vi "PartSetup.vi"(8 "error in (no error)":errorcluster) -> (0 "error out":errorcluster)   [LabVIEW 2015]
uses:
  Control 1.ctl
  Partsetup-Exit.ctl
  Partsetup-Delete.ctl
  Partsetup- Save.ctl
  <vilib>/addons/database/_DB Variant To Data/Database Variant To Data.xnode
  <vilib>/addons/database/NI_Database_API.lvlib
  <vilib>/addons/database/Connection.llb/DB Tools Open Connec (String).vi
  Galobal variable_TI.vi
panel:
  in  "Save":T1
  in  "Delete":T2
  in  "Exit":T3
  in  "Data Insert":variant
  in  "Existing Model Name":string(combo)
  in  "Part setup":T4
  # "UM"
  # "Atma Autotech Engineers Pvt.Ltd"
  # "PART SETUP"
  # "Existing Model Name"
  # "First motor testing Parameter"
  # "Printing Info"
  # "Second motor testing Parameter"
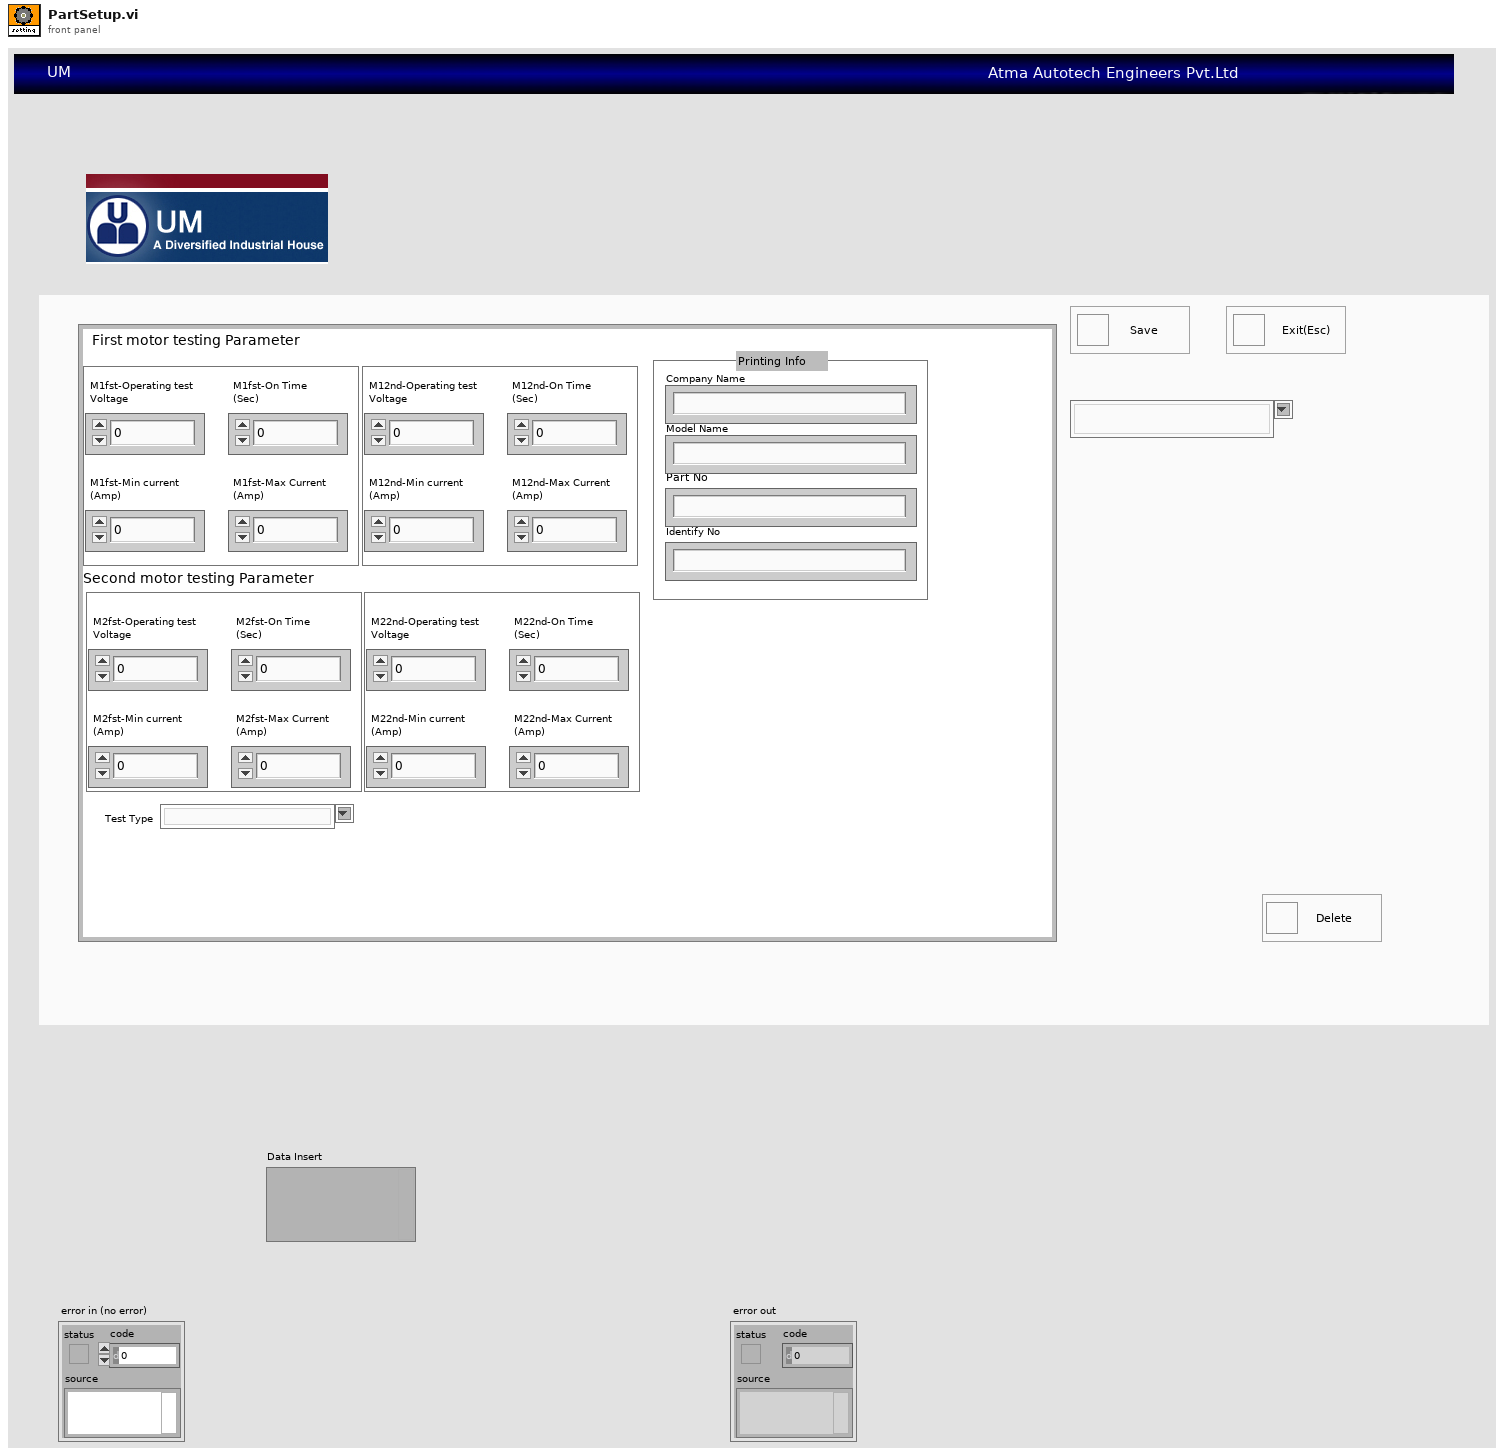
[diagram p1: front panel]
types:
  T1 = typedef "Partsetup- Save.ctl" = bool
  T2 = typedef "Partsetup-Delete.ctl" = bool
  T3 = typedef "Partsetup-Exit.ctl" = bool
  T4 = typedef "Control 1.ctl" = cluster{"Model Name":string, "Company Name":string, "Part No":string, "Identify No":string, "M1fst-Operating test\nVoltage":dbl, "M1fst-On Time \n(Sec)":dbl, "M1fst-Min current \n(Amp)":dbl, "M1fst-Max Current\n(Amp)":dbl, "M12nd-Operating test\nVoltage":dbl, "M12nd-On Time \n(Sec)":dbl, "M12nd-Min current \n(Amp)":dbl, "M12nd-Max Current\n(Amp)":dbl, "M2fst-Operating test\nVoltage":dbl, "M2fst-On Time \n(Sec)":dbl, "M2fst-Min current \n(Amp)":dbl, "M2fst-Max Current\n(Amp)":dbl, "M22nd-Operating test\nVoltage":dbl, "M22nd-On Time \n(Sec)":dbl, "M22nd-Min current \n(Amp)":dbl, "M22nd-Max Current\n(Amp)":dbl, "Test Type ":string}
  T5 = enum16{"New model Create", "Update", "DB-Read by condition", "DB-Read", "Delete"}
  T6 = typedef "NI_Database_API.lvlib/Conn ObjectReference.ctl" = refnum<k1>
  T7 = enum16{"Left Button", "Center Button", "Right Button", "Window Close"}
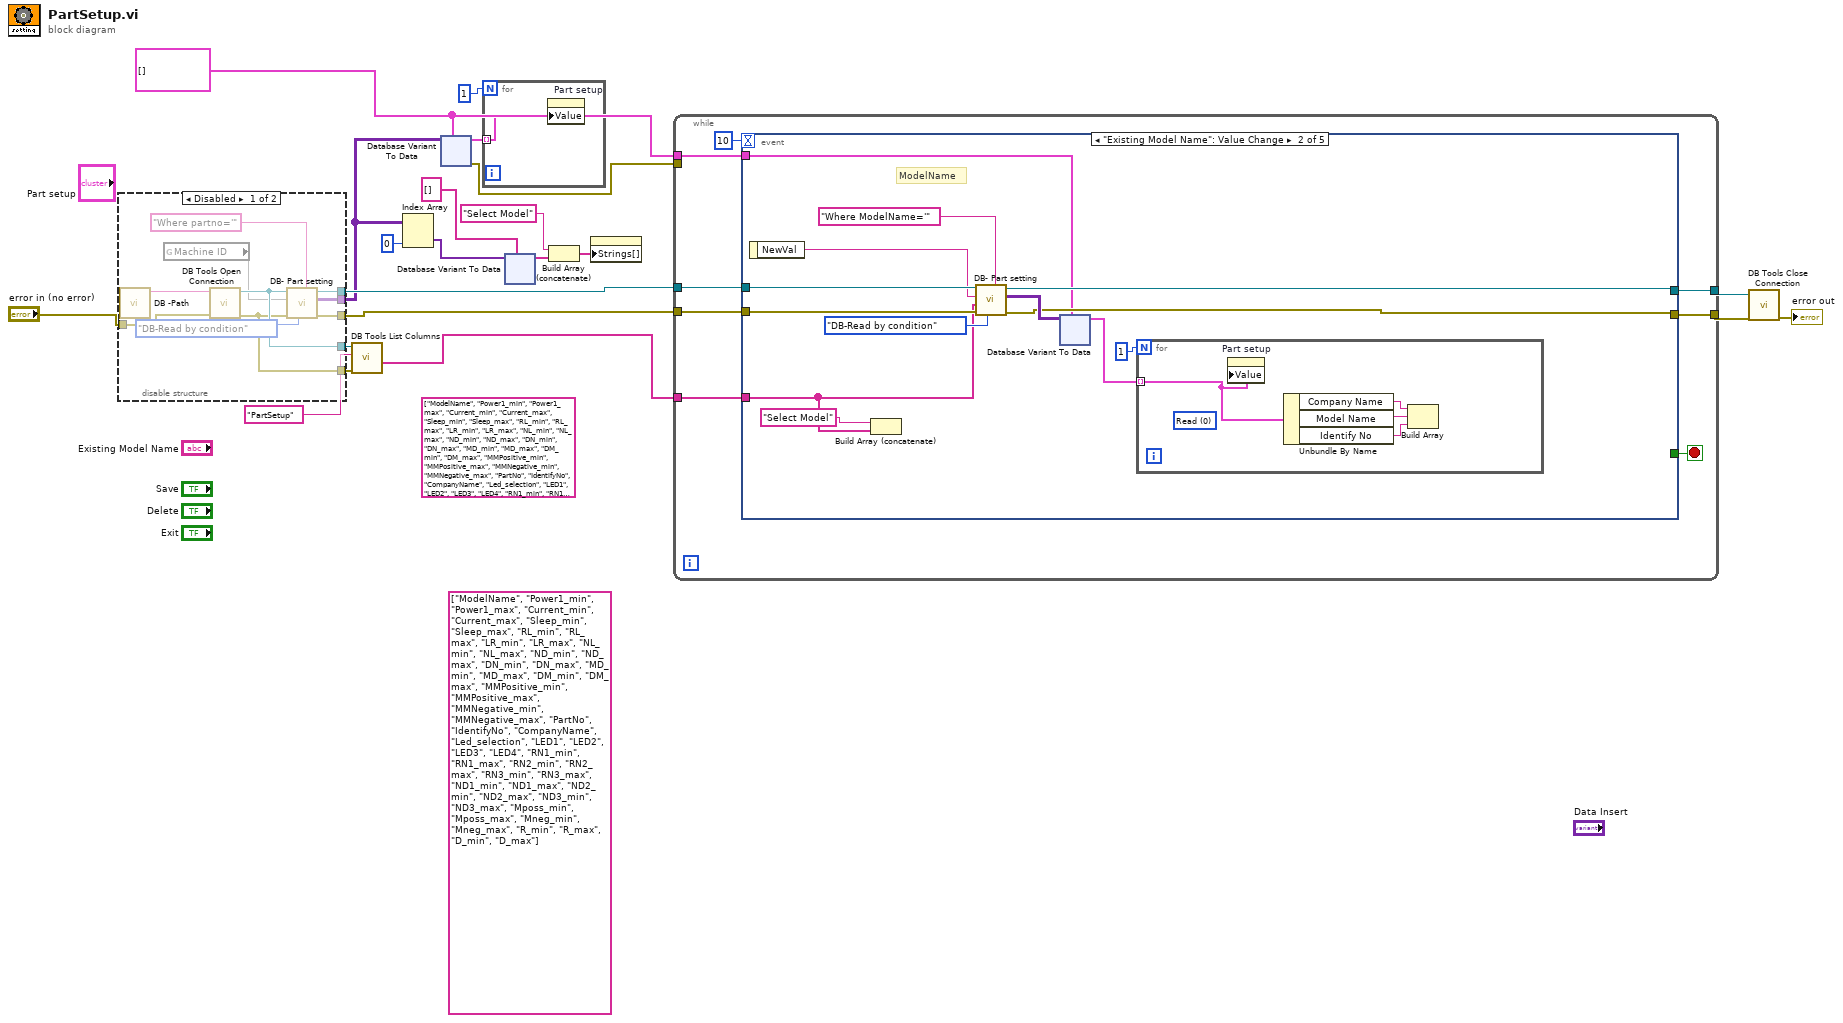
[diagram p0: block diagram]
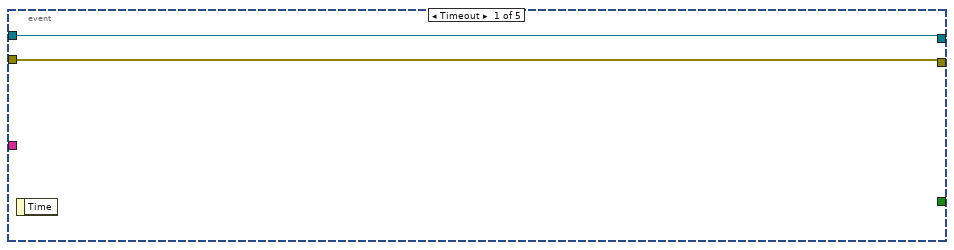
[diagram p3: hidden frame]
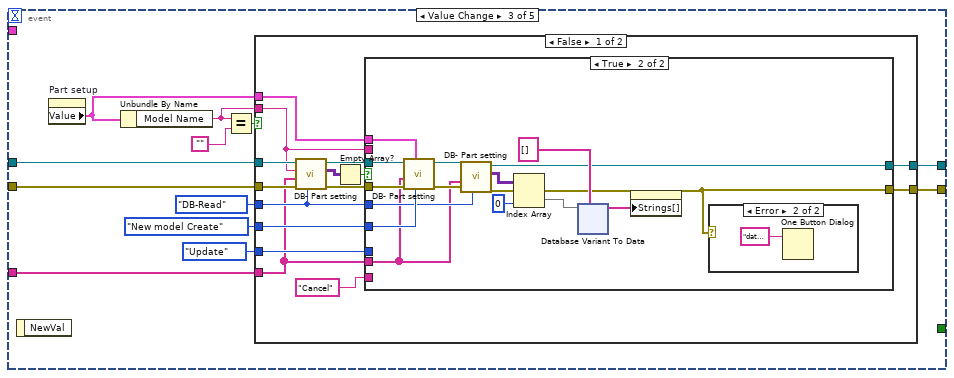
[diagram p4: hidden frame]
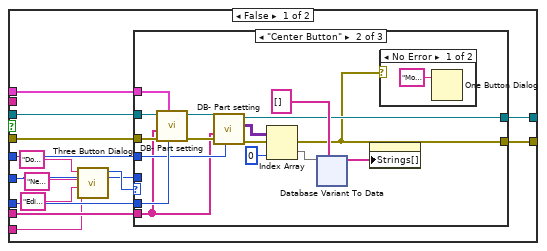
[diagram p5: hidden frame]
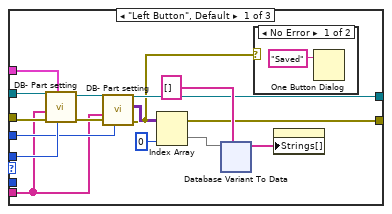
[diagram p6: hidden frame]
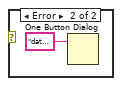
[diagram p7: hidden frame]
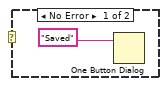
[diagram p10: hidden frame]
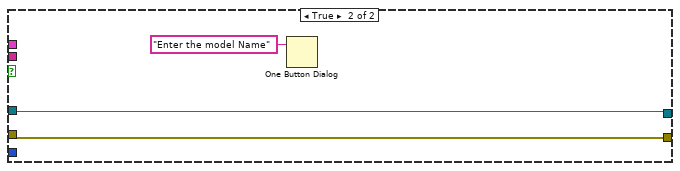
[diagram p11: hidden frame]
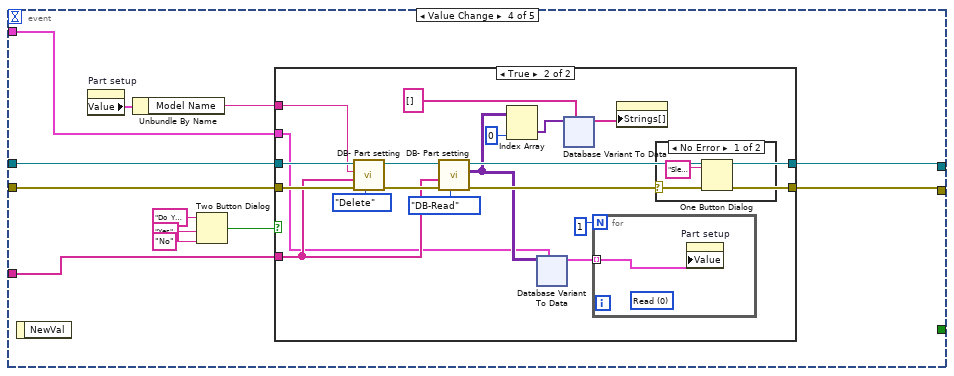
[diagram p12: hidden frame]
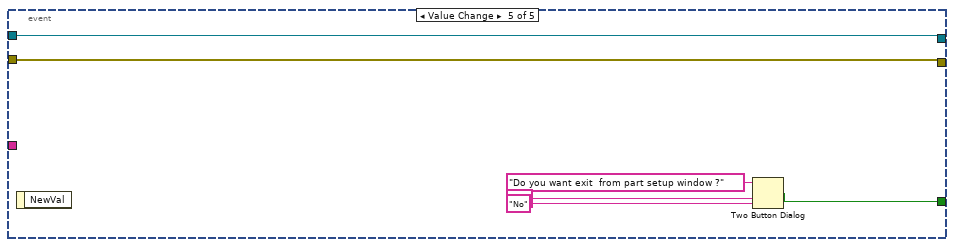
[diagram p15: hidden frame]
diagram:
  w4 = T4[] []
  (unwired) string[] ["ModelName", "Power1_min", "Power1_max", "Current_min", "Current_max", "Sleep_min", "Sleep_max", "RL_min", "RL_max", "LR_min", "LR_max", "NL_min", "NL_max", "ND_min", "ND_max", "DN_min", "DN_max", "MD_min", "MD_max", "DM_min", "DM_max", "MMPositive_min", "MMPositive_max", "MMNegative_min", "MMNegative_max", "PartNo", "IdentifyNo", "CompanyName", "Led_selection", "LED1", "LED2", "LED3", "LED4", "RN1_min", "RN1_max", "RN3_min", "RN3_max", "ND1_min", "ND1_max", "ND2_min", "ND2_max", "Mposs_min", "Mposs_max", "Mneg_min", "Mneg_max", "R_min", "R_max", "D_min", "D_max"] ("columns")
  (unwired) string[] ["ModelName", "Power1_min", "Power1_max", "Current_min", "Current_max", "Sleep_min", "Sleep_max", "RL_min", "RL_max", "LR_min", "LR_max", "NL_min", "NL_max", "ND_min", "ND_max", "DN_min", "DN_max", "MD_min", "MD_max", "DM_min", "DM_max", "MMPositive_min", "MMPositive_max", "MMNegative_min", "MMNegative_max", "PartNo", "IdentifyNo", "CompanyName", "Led_selection", "LED1", "LED2", "LED3", "LED4", "RN1_min", "RN1_max", "RN2_min", "RN2_max", "RN3_min", "RN3_max", "ND1_min", "ND1_max", "ND2_min", "ND2_max", "ND3_min", "ND3_max", "Mposs_min", "Mposs_max", "Mneg_min", "Mneg_max", "R_min", "R_max", "D_min", "D_max"] ("columnsName")
  n1 = disable-structure shown="Disabled" {
    disable-tunnel: "error in (no error)" -> [w30 _]
    disable-tunnel: [w29 _] -> w18
    disable-tunnel: [w28 _] -> w17
    disable-tunnel: [w26 _] -> w11
    disable-tunnel: [w25 _] -> w8
    disable-tunnel: [w24 _] -> w7
    frame Disabled {
      n2 = call "DB -Path.vi"() -> ("String"=w31:string)  [unwired: 11 in]
      n3 = global read "Galobal variable_TI.vi" "Machine ID"() -> (w23)
      n4 = call-poly <vilib>:"DB Tools Open Connection.vi"("error in (no error)"=w30, "connection information"=w31) -> ("error out"=w24:errorcluster, "connection reference"=w25:T6)  [unwired: 6 in]
      n5 = call "DB- Part setting.vi"("string"="Where partno='", "Enum"=T5."DB-Read by condition", "error in (no error)"=w24, "Model Name"=w23, "connection reference"=w25) -> ("error out"=w28:errorcluster, "Data Read"=w26:variant[][], "Refnum out"=w29:T6)  [unwired: 4 in]
    }
    frame Enabled {
    }
  }
  n6 = call <vilib>:"DB Tools List Columns.vi"("error in (no error)"=w7, "table"="PartSetup", "connection reference"=w8) -> ("columns"=w5:string[])  [unwired: 1 in, 3 out]
  n7 = Index Array(array=w11, index (col)=0 ("disabled index (col)")) -> (element=w15:variant[])  [unwired: 1 in]
  n8 = xnode "Database Variant To Data"("database variant"=w11, "type"=w4) -> ("data"=w12:T4[], "error out"=w10:errorcluster)  [unwired: 1 in]
  n9 = for {
    N: 1 -> [_]
    tunnel: w12 -> [w32] mode=indexing
    n10 = property on="Part setup" class="Clust (strict)"("Value"=w32) -> ()  [unwired: 2 in, 2 out]
  }
  n11 = xnode "Database Variant To Data"("database variant"=w15, "type"=string[] []) -> ("data"=w2:string[])  [unwired: 1 in, 1 out]
  n12 = Build Array (concatenate)("Select Model", w2) -> (w3:string[])
  n13 = property on="Existing Model Name" class="CmbBox"("Strings[]"=w3) -> ()  [unwired: 2 in, 2 out]
  n14 = while {
    tunnel: w18 -> [w40]
    tunnel: w17 -> [w39]
    tunnel: [w38] -> w21
    tunnel: [w37] -> w20
    tunnel: w5 -> [w35]
    tunnel: w10 -> [_]
    tunnel: w4 -> [w34]
    stop <- w36 stop-if-true
    n15 = event shown="[1] \"Existing Model Name\": Value Change" {
      selector: _ -> [_ _ _ _ _]
      dyn-events: _ -> [_ _ _ _ _]
      timeout: 10 -> [_ _ _ _ _]
      tunnel: w40 -> [w42 w55 w730 w941 w1665]
      tunnel: w39 -> [w41 w54 w722 w940 w1664]
      tunnel: [w41 w48 w725 w933 w1664] -> w37
      tunnel: [w42 w49 w724 w934 w1665] -> w38
      tunnel: [_ _ _ _ w1666] -> w36
      tunnel: w35 -> [_ w46 w723 w932 _]
      tunnel: w34 -> [_ w47 _ w931 _]
      event Timeout {
        n16 = event-data() -> ()  [unwired: 1 in, 1 out]
      }
      event "Existing Model Name": Value Change {
        # "ModelName"
        n17 = event-data() -> ("NewVal"=w44:string)  [unwired: 1 in]
        n18 = Build Array (concatenate)("Select Model", w46) -> ()  [unwired: 1 out]
        n19 = call "DB- Part setting.vi"("string"="Where ModelName='", "Enum"=T5."DB-Read by condition", "error in (no error)"=w54, "columnsName"=w46, "Model Name"=w44, "connection reference"=w55) -> ("error out"=w48:errorcluster, "Data Read"=w52:variant[][], "Refnum out"=w49:T6)  [unwired: 3 in]
        n20 = xnode "Database Variant To Data"("database variant"=w52, "type"=w47) -> ("data"=w51:T4[])  [unwired: 1 in, 1 out]
        n21 = for {
          N: 1 -> [_]
          tunnel: w51 -> [w56] mode=indexing
          (unwired) u16 0 items=["Read", "Write"] ("read/write")
          n22 = property on="Part setup" class="Clust (strict)"("Value"=w56) -> ()  [unwired: 2 in, 2 out]
          n23 = Unbundle By Name(w56) -> ("Company Name"=w59:string, "Model Name"=w58:string, "Identify No"=w57:string)
          n24 = Build Array(w59, w58, w57) -> ()  [unwired: 1 out]
        }
      }
      event Value Change {
        n25 = event-data() -> ()  [unwired: 1 in, 1 out]
        n26 = property on="Part setup" class="Clust (strict)"() -> ("Value"=w721:T4)  [unwired: 2 in, 2 out]
        n27 = Unbundle By Name(w721) -> ("Model Name"=w728:string)
        n28 = Equal?(x=w728, y="") -> (x = y?=w731:bool)
        n29 = case shown="False" w731 {
          tunnel: w730 -> [w747 w929]
          tunnel: w722 -> [w746 w928]
          tunnel: T5."DB-Read" ("Enum") -> [w738 _]
          tunnel: w728 -> [w735 _]
          tunnel: w721 -> [w741 _]
          tunnel: T5."New model Create" ("Enum") -> [w740 _]
          tunnel: T5."Update" ("Enum") -> [w739 _]
          tunnel: [w737 w928] -> w725
          tunnel: [w736 w929] -> w724
          tunnel: w723 -> [w734 _]
          frame False {
            n30 = call "DB- Part setting.vi"("Enum"=w738, "error in (no error)"=w746, "columnsName"=w734, "Model Name"=w735, "connection reference"=w747) -> ("error out"=w742:errorcluster, "Data Read"=w745:variant[][], "Refnum out"=w743:T6)  [unwired: 4 in]
            n31 = Empty Array?(array=w745) -> (empty?=w744:bool)
            n32 = case shown="True" w744 {
              tunnel: w743 -> [w761 w887]
              tunnel: w742 -> [w760 w886]
              tunnel: w741 -> [w748 w885]
              tunnel: w740 -> [w749 w884]
              tunnel: w739 -> [w759 _]
              tunnel: w738 -> [w755 w881]
              tunnel: [w756 w874] -> w737
              tunnel: [w757 w876] -> w736
              tunnel: w735 -> [_ _]
              tunnel: w734 -> [w754 w875]
              tunnel: "Cancel" ("F button name (\"Cancel\")") -> [w750 _]
              frame False {
                n33 = call <vilib>:"Three Button Dialog.vi"("Right Button Text (\"Cancel\")"=w750, "Center Button Text (\"No\")"="Edit Model Name" ("F button name (\"Cancel\")"), "Left Button Text (\"Yes\")"="New Model Create" ("T button name (\"OK\")"), "message"="Do you want modification Or New Create Model Name ?") -> ("Which Button?"=w758:T7)  [unwired: 7 in]
                n34 = case shown="\"Center Button\"" w758 {
                  tunnel: w761 -> [w774 w825 w872]
                  tunnel: w760 -> [w773 w824 w871]
                  tunnel: w759 -> [_ w823 _]
                  tunnel: [w766 w822 w872] -> w757
                  tunnel: [w765 w819 w871] -> w756
                  tunnel: w755 -> [w771 w821 _]
                  tunnel: w754 -> [w763 w820 _]
                  tunnel: w749 -> [w772 _ _]
                  tunnel: w748 -> [w764 w818 _]
                  frame "Left Button", Default {
                    n35 = call "DB- Part setting.vi"("Enum"=w772, "Data Insert"=w764, "error in (no error)"=w773, "columnsName"=w763, "connection reference"=w774) -> ("error out"=w776:errorcluster, "Refnum out"=w775:T6)  [unwired: 4 in, 1 out]
                    n36 = call "DB- Part setting.vi"("Enum"=w771, "error in (no error)"=w776, "columnsName"=w763, "connection reference"=w775) -> ("error out"=w765:errorcluster, "Data Read"=w767:variant[][], "Refnum out"=w766:T6)  [unwired: 5 in]
                    n37 = Index Array(array=w767, index (col)=0 ("disabled index (col)")) -> (element=w770:variant[])  [unwired: 1 in]
                    n38 = xnode "Database Variant To Data"("database variant"=w770, "type"=string[] []) -> ("data"=w762:string[])  [unwired: 1 in, 1 out]
                    n39 = case shown="No Error" w765 {
                      frame No Error {
                        n40 = One Button Dialog(message="Saved") -> ()  [unwired: 1 in, 1 out]
                      }
                      frame Error {
                        n41 = One Button Dialog(message="data not saved") -> ()  [unwired: 1 in, 1 out]
                      }
                    }
                    n42 = property on="Existing Model Name" class="CmbBox"("Strings[]"=w762) -> ()  [unwired: 2 in, 2 out]
                  }
                  frame "Center Button" {
                    n43 = call "DB- Part setting.vi"("Enum"=w823, "Data Insert"=w818, "error in (no error)"=w824, "columnsName"=w820, "connection reference"=w825) -> ("error out"=w831:errorcluster, "Refnum out"=w830:T6)  [unwired: 4 in, 1 out]
                    n44 = call "DB- Part setting.vi"("Enum"=w821, "error in (no error)"=w831, "columnsName"=w820, "connection reference"=w830) -> ("error out"=w819:errorcluster, "Data Read"=w829:variant[][], "Refnum out"=w822:T6)  [unwired: 5 in]
                    n45 = Index Array(array=w829, index (col)=0 ("disabled index (col)")) -> (element=w828:variant[])  [unwired: 1 in]
                    n46 = xnode "Database Variant To Data"("database variant"=w828, "type"=string[] []) -> ("data"=w817:string[])  [unwired: 1 in, 1 out]
                    n47 = property on="Existing Model Name" class="CmbBox"("Strings[]"=w817) -> ()  [unwired: 2 in, 2 out]
                    n48 = case shown="No Error" w819 {
                      frame No Error {
                        n49 = One Button Dialog(message="Modified data save") -> ()  [unwired: 1 in, 1 out]
                      }
                      frame Error {
                      }
                    }
                  }
                  frame "Right Button" {
                  }
                }
              }
              frame True {
                n50 = call "DB- Part setting.vi"("Enum"=w884, "Data Insert"=w885, "error in (no error)"=w886, "columnsName"=w875, "connection reference"=w887) -> ("error out"=w883:errorcluster, "Refnum out"=w882:T6)  [unwired: 4 in, 1 out]
                n51 = call "DB- Part setting.vi"("Enum"=w881, "error in (no error)"=w883, "columnsName"=w875, "connection reference"=w882) -> ("error out"=w874:errorcluster, "Data Read"=w880:variant[][], "Refnum out"=w876:T6)  [unwired: 5 in]
                n52 = Index Array(array=w880, index (col)=0 ("disabled index (col)")) -> (element=w879:variant[])  [unwired: 1 in]
                n53 = xnode "Database Variant To Data"("database variant"=w879, "type"=string[] []) -> ("data"=w873:string[])  [unwired: 1 in, 1 out]
                n54 = property on="Existing Model Name" class="CmbBox"("Strings[]"=w873) -> ()  [unwired: 2 in, 2 out]
                n55 = case shown="Error" w874 {
                  frame No Error {
                    n56 = One Button Dialog(message="Saved") -> ()  [unwired: 1 in, 1 out]
                  }
                  frame Error {
                    n57 = One Button Dialog(message="data not saved") -> ()  [unwired: 1 in, 1 out]
                  }
                }
              }
            }
          }
          frame True {
            n58 = One Button Dialog(message="Enter the model Name") -> ()  [unwired: 1 in, 1 out]
          }
        }
      }
      event Value Change {
        n59 = event-data() -> ()  [unwired: 1 in, 1 out]
        n60 = property on="Part setup" class="Clust (strict)"() -> ("Value"=w942:T4)  [unwired: 2 in, 2 out]
        n61 = Unbundle By Name(w942) -> ("Model Name"=w935:string)
        n62 = Two Button Dialog(message="Do  You Want Delete The Existing Model Name ?", 1:"No" ("T button name (\"OK\")"), 2:"Yes" ("T button name (\"OK\")")) -> (T button?=w936:bool)
        n63 = case shown="True" w936 {
          tunnel: w941 -> [w944 w962]
          tunnel: w940 -> [w943 w961]
          tunnel: w935 -> [_ w960]
          tunnel: [w944 w955] -> w934
          tunnel: [w943 w954] -> w933
          tunnel: w932 -> [_ w953]
          tunnel: w931 -> [_ w946]
          frame False {
          }
          frame True {
            n64 = call "DB- Part setting.vi"("Enum"=T5."Delete", "error in (no error)"=w961, "columnsName"=w953, "Model Name"=w960, "connection reference"=w962) -> ("error out"=w959:errorcluster, "Refnum out"=w956:T6)  [unwired: 4 in, 1 out]
            n65 = call "DB- Part setting.vi"("Enum"=T5."DB-Read", "error in (no error)"=w959, "columnsName"=w953, "connection reference"=w956) -> ("error out"=w954:errorcluster, "Data Read"=w951:variant[][], "Refnum out"=w955:T6)  [unwired: 5 in]
            n66 = Index Array(array=w951, index (col)=0 ("disabled index (col)")) -> (element=w949:variant[])  [unwired: 1 in]
            n67 = xnode "Database Variant To Data"("database variant"=w951, "type"=w946) -> ("data"=w947:T4[])  [unwired: 1 in, 1 out]
            n68 = xnode "Database Variant To Data"("database variant"=w949, "type"=string[] []) -> ("data"=w945:string[])  [unwired: 1 in, 1 out]
            n69 = for {
              N: 1 -> [_]
              tunnel: w947 -> [w1001] mode=indexing
              (unwired) u16 0 items=["Read", "Write"] ("read/write")
              n70 = property on="Part setup" class="Clust (strict)"("Value"=w1001) -> ()  [unwired: 2 in, 2 out]
            }
            n71 = property on="Existing Model Name" class="CmbBox"("Strings[]"=w945) -> ()  [unwired: 2 in, 2 out]
            n72 = case shown="No Error" w954 {
              frame No Error {
                n73 = One Button Dialog(message="Slected existing model name has been deleted" ("T button name (\"OK\")")) -> ()  [unwired: 1 in, 1 out]
              }
              frame Error {
              }
            }
          }
        }
      }
      event Value Change {
        n74 = event-data() -> ()  [unwired: 1 in, 1 out]
        n75 = Two Button Dialog(message="Do you want exit  from part setup window ?", 1:"No" ("T button name (\"OK\")"), 2:"Yes" ("T button name (\"OK\")")) -> (T button?=w1666:bool)
      }
    }
  }
  n76 = call <vilib>:"DB Tools Close Connection.vi"("error in (no error)"=w20, "connection reference"=w21) -> ("error out"=→"error out":errorcluster)  [unwired: 5 in]
